vi "shag_start — 11.vi"() -> ()   [LabVIEW 2016]
uses:
  <vilib>/Instr/_visa.llb/VISA Configure Serial Port (Instr).vi
panel:
  out "положение в мин 4":i32
  out "text4":string
  out "4":i32
  out "3":i32
  out "положение в мин 3":i32
  out "text3":string
  out "text":string
  out "2":i32
  out "1":i32
  out "text2":string
  out "положение в мин 2":i32
  out "положение в мин 1":i32
  in  "all":T1(tab)
  out "положение шд 2":i32(knob) scale=-10.0..190.0
  out "текущее положение 2":string
  out "положение в минутах 2":string
  in  "Минуты 2":i32 min=-600 max=11400
  in  "Stop двигатель 2":bool
  in  "Вращение по градусам +  2":bool
  in  "Вращение по градусам -  2":bool
  in  "Вернуться в нулевое положение 2":bool
  in  "Задать текущее положение нулевым 2":bool
  in  "Установка минут 2":bool
  in  "Блокировать трубку №2":bool
  out "положение шд":i32(knob) scale=-10.0..190.0
  out "градусы минуты":string
  out "минуты":string
  in  "Минуты":i32 min=-600 max=11400
  in  "Stop двигатель":bool
  in  "Вращение по градусам +":bool
  in  "Вращение по градусам -":bool
  in  "Вернуться в нулевое положение":bool
  in  "Задать текущее положение нулевым":bool
  in  "Установка минут":bool
  in  "Блокировать зеркало №1":bool
  in  "stop":bool
  out "положение шд 3":i32(knob) scale=-10.0..190.0
  out "текущее положение 3":string
  out "положение в минутах 3":string
  in  "Минуты 3":i32 min=-600 max=11400
  in  "Stop двигатель 3":bool
  in  "Вращение по градусам +  3":bool
  in  "Вращение по градусам -  3":bool
  in  "Вернуться в нулевое положение 3":bool
  in  "Задать текущее положение нулевым 3":bool
  in  "Установка минут 3":bool
  in  "Блокировать стол №3":bool caption="Блокировать трубку №2"
  out "положение шд 4":i32(knob) scale=-10.0..190.0
  out "текущее положение 4":string
  out "положение в минутах 4":string
  in  "Минуты 4":i32 min=-600 max=11400
  in  "Stop двигатель 4":bool
  in  "Вращение по градусам +  4":bool
  in  "Вращение по градусам -  4":bool
  in  "Вернуться в нулевое положение 4":bool
  in  "Задать текущее положение нулевым 4":bool
  in  "Установка минут 4":bool
  in  "Блокировать стол №3 2":bool caption="Блокировать трубку №2"
  in  "Выберете COM порт":refnum<visa-resource-name>="COM1"
  in  "Скорость обмена данными":u32(ring)=19200 items=["9600"=9600, "19200"=19200, "38400"=38400, "57600"=57600]
  in  "Число бит на символ":u16=8 min=5 max=8 step=1
  in  "Контроль чётности":enum16{"None", "Odd", "Even", "Mark", "Space"}(ring)
  in  "Стоповый бит":u16(ring)=10 items=["1.0"=10, "1.5"=15, "2.0"=20]
  in  "Контроль переполнения":u16(ring) items=["None"=0, "XON/XOFF"=1, "RTS/CTS"=2, "DTR/DSR"=4]
  # "1 - адресс 1 двигателя\n2 - адресс 2 двигателя\n$0MV\\01+   - запуск всех двигателей в положительном направлении \n$0MS\\00   - остановка всех двигателей\n$0MJ\\04+\\00\\00\\01   - 1 шаг всех двигателей\n$0SS\\01\\10   - скорость 10 для всех двигателей"
  # "Зеркало №1"
  # "Текущее положение:"
  # "Ренгеновская трубка №2"
  # "Положение:"
  # "Поворотный стол №3"
  # "Положение:"
  # "Счётчик №4"
  # "Положение:"
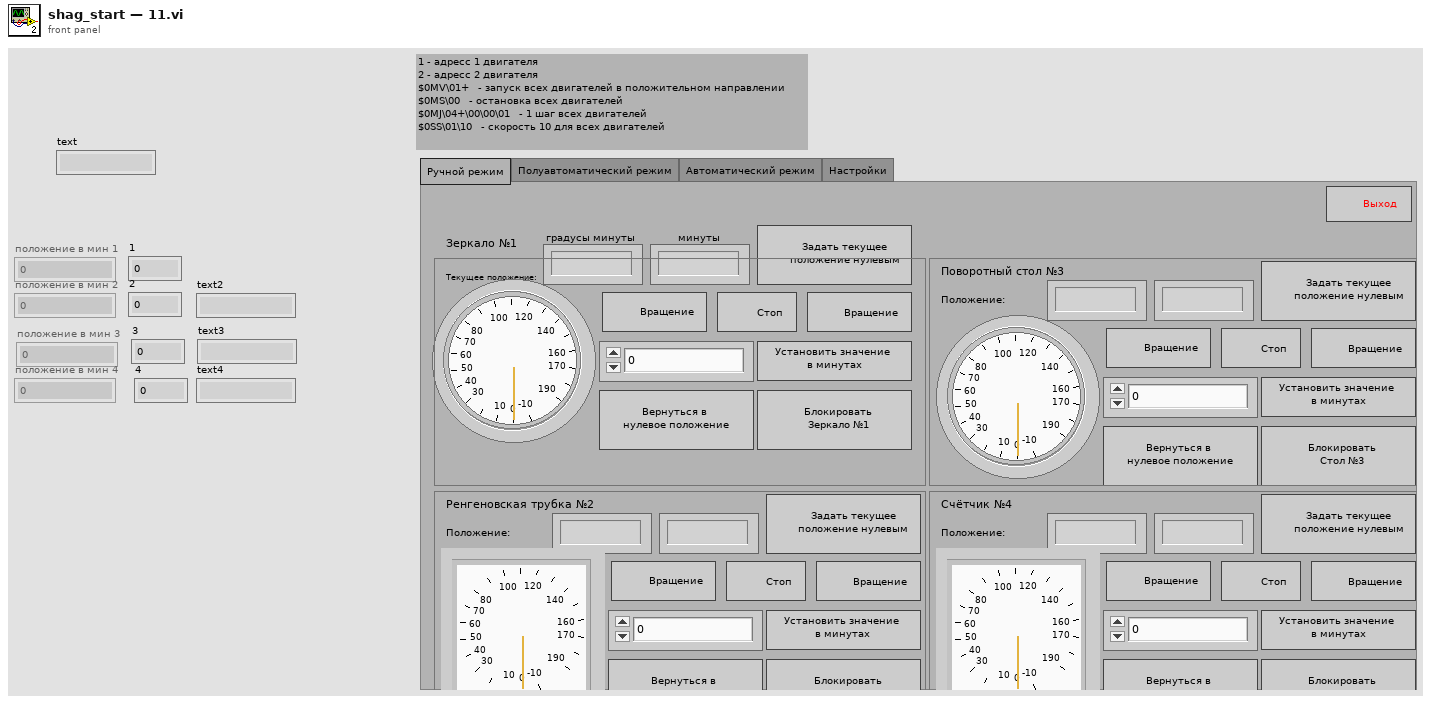
[diagram p1: front panel]
types:
  T1 = enum32{"Ручной режим", "Полуавтоматический режим", "Автоматический режим", "Настройки"}
  T2 = enum16{"open", "replace", "create", "open or create", "replace or create", "replace or create with confirmation"}
  T3 = enum8{"Enabled", "Disabled", "Disabled and Grayed Out"}
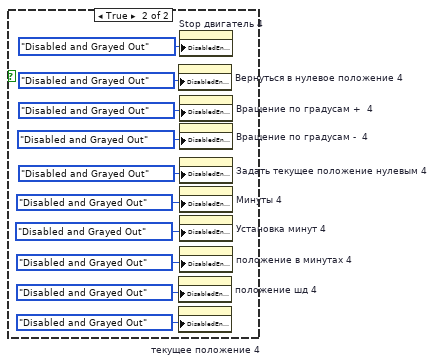
[diagram p2: hidden frame]
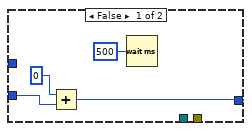
[diagram p4: hidden frame]
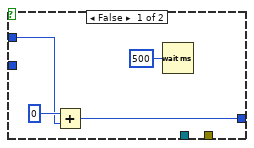
[diagram p5: hidden frame]
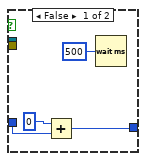
[diagram p6: hidden frame]
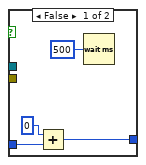
[diagram p7: hidden frame]
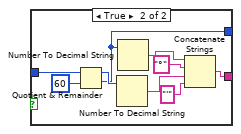
[diagram p8: hidden frame]
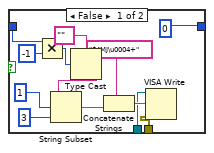
[diagram p10: hidden frame]
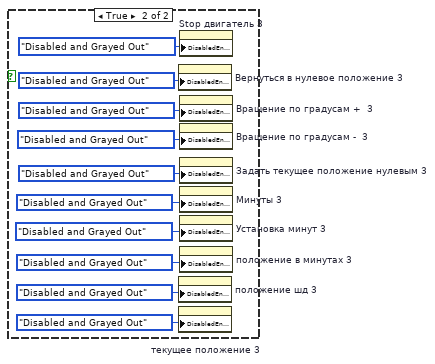
[diagram p13: hidden frame]
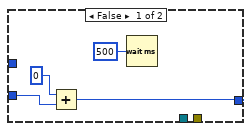
[diagram p16: hidden frame]
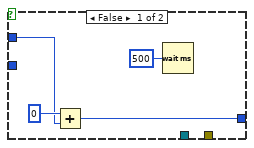
[diagram p17: hidden frame]
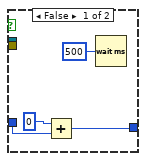
[diagram p18: hidden frame]
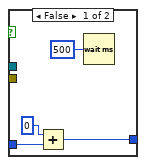
[diagram p19: hidden frame]
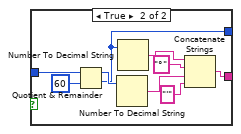
[diagram p20: hidden frame]
diagram:
  n1 = call-poly "VISA Configure Serial Port"("VISA resource name"="Выберете COM порт", "baud rate (9600)"="Скорость обмена данными", "data bits (8)"="Число бит на символ", "parity (0:none)"="Контроль чётности", "stop bits (10: 1 bit)"="Стоповый бит", "flow control (0:none)"="Контроль переполнения") -> ("VISA resource name out"=w32:refnum<visa-resource-name>, "error out"=w31:errorcluster)  [unwired: 8 in]
  n2 = Boolean To (0,1)(Boolean=FALSE ("DTR Write")) -> (0, 1=w33:i16)
  n3 = Boolean To (0,1)(Boolean=FALSE ("DTR Write")) -> (0, 1=w34:i16)
  n4 = property class="Instr"(reference=w32, error in=w31, "Serial Settings:Modem Line Settings:Line DTR State"=w33, "Serial Settings:Modem Line Settings:Line RTS State"=w34) -> (reference out=w30:refnum<visa-resource-name>, error out=w29:errorcluster)
  n5 = flat-sequence {
    tunnel: w30 -> [w63]
    tunnel: w29 -> [w62]
    tunnel: [w63] -> w28
    tunnel: [w62] -> w27
    tunnel: [w58] -> w18
    tunnel: [w66] -> w17
    tunnel: w28 -> [w66]
    tunnel: w27 -> [w65]
    tunnel: [w65] -> w15
    tunnel: [w66] -> w13
    tunnel: [w65] -> w11
    tunnel: w18 -> [w67]
    tunnel: [w65] -> w6
    tunnel: [w66] -> w5
    tunnel: [w66] -> w3
    tunnel: [w65] -> w1
    tunnel: w17 -> [w80]
    tunnel: [w80] -> w16
    tunnel: w15 -> [w79]
    tunnel: [w79] -> w14
    tunnel: w13 -> [w72]
    tunnel: [w72] -> w12
    tunnel: w11 -> [w74]
    tunnel: [w74] -> w10
    tunnel: [w75] -> w9
    tunnel: [w73] -> w8
    tunnel: [w71] -> w7
    tunnel: w6 -> [w73]
    tunnel: w5 -> [w71]
    tunnel: [w70] -> w4
    tunnel: w3 -> [w70]
    tunnel: [w69] -> w2
    tunnel: w1 -> [w69]
    tunnel: w16 -> [w90]
    tunnel: w14 -> [w89]
    tunnel: w12 -> [w85]
    tunnel: w10 -> [w88]
    tunnel: w9 -> [w87]
    tunnel: w8 -> [w84]
    tunnel: w7 -> [w83]
    tunnel: w4 -> [w82]
    tunnel: w2 -> [w81]
    frame #0 {
      n6 = VISA Write(VISA resource name=w63, write buffer="$0SS\u0001\u0010", error in (no error)=w62) -> ()  [unwired: 3 out]
      n7 = Open/Create/Replace File(file path (use dialog)=path "C:/Users/User/Desktop/shagovi_dvigatel/test_text_file", operation (0:open)=T2."open", access (0:read/write)=enum16{"read/write", "read-only", "write-only"}."read-only") -> (refnum out=w57:refnum<file>)  [unwired: 3 in, 2 out]
      n8 = Read from Text File(file (use dialog)=w57) -> (refnum out=w58:refnum<file>, text=w44:string)  [unwired: 3 in, 2 out]
      "text" <- w44
      n9 = Spreadsheet String To Array(delimiter (Tab)=" ", format string="%5f", spreadsheet string=w44) -> (array=w54:dbl[][])  [unwired: 1 in]
      n10 = Index Array(array=w54, index (row)=0 ("index")) -> (element=w52:dbl[])  [unwired: 1 in]
      n11 = Decimate 1D Array(w52) -> (w49:dbl[], w40:dbl[], w39:dbl[], w35:dbl[])
      n12 = Index Array(array=w35, index=0) -> (element=w37:dbl)
      n13 = Index Array(array=w39, index=0) -> (element=w42:dbl)
      n14 = Index Array(array=w40, index=0) -> (element=w48:dbl)
      n15 = To Long Integer(number=w37) -> (32bit integer=→"4":i32)
      n16 = To Long Integer(number=w42) -> (32bit integer=→"3":i32)
      n17 = Index Array(array=w49, index=0) -> (element=w47:dbl)
      n18 = To Long Integer(number=w48) -> (32bit integer=→"2":i32)
      n19 = To Long Integer(number=w47) -> (32bit integer=→"1":i32)
    }
    frame #1 {
      n20 = Close File(refnum=w67) -> ()  [unwired: 1 in, 2 out]
      n21 = Wait (ms)(milliseconds to wait=u32 500) -> ()  [unwired: 1 out]
    }
    frame #2 {
      n22 = Open/Create/Replace File(file path (use dialog)=path "C:/Users/User/Desktop/shagovi_dvigatel/test_text_file", operation (0:open)=T2."replace or create", access (0:read/write)=enum16{"read/write", "read-only", "write-only"}."write-only") -> (refnum out=w75:refnum<file>)  [unwired: 3 in, 2 out]
    }
    frame #3 {
      n23 = while {
        tunnel: w90 -> [w221]
        tunnel: w89 -> [w220]
        shift-right: [w216] -> _
        shift-left: _ -> [w225]
        shift-right: [w217] -> _
        shift-left: _ -> [w224]
        shift-right: [w218] -> _
        shift-left: _ -> [w223]
        shift-right: [w219] -> _
        shift-left: _ -> [w222]
        tunnel: w88 -> [w190]
        shift-right: [w212] -> w86
        shift-left: w87 -> [w213]
        tunnel: w85 -> [w189]
        shift-right: [w185] -> _
        shift-left: _ -> [w186]
        shift-right: [w183] -> _
        shift-left: _ -> [w184]
        shift-right: [w181] -> _
        shift-left: _ -> [w182]
        shift-right: [w179] -> _
        shift-left: _ -> [w180]
        tunnel: w84 -> [w157]
        tunnel: w83 -> [w156]
        shift-right: [w153] -> _
        shift-left: _ -> [w154]
        shift-right: [w151] -> _
        shift-left: _ -> [w152]
        shift-right: [w149] -> _
        shift-left: _ -> [w150]
        shift-right: [w147] -> _
        shift-left: _ -> [w148]
        tunnel: w82 -> [w125]
        tunnel: w81 -> [w124]
        shift-right: [w121] -> _
        shift-left: _ -> [w122]
        shift-right: [w119] -> _
        shift-left: _ -> [w120]
        shift-right: [w117] -> _
        shift-left: _ -> [w118]
        shift-right: [w115] -> _
        shift-left: _ -> [w116]
        stop <- "stop" stop-if-true
        # "Остановка двигателя"
        # "Управление вращением"
        # "Управление вращением"
        n24 = flat-sequence {
          tunnel: w157 -> [w549]
          tunnel: w156 -> [w548]
          tunnel: [w548] -> w178
          tunnel: [w549] -> w177
          tunnel: ["Вращение по градусам +  3"] -> w176
          tunnel: ["Вращение по градусам -  3"] -> w175
          tunnel: ["Вернуться в нулевое положение 3"] -> w174
          tunnel: ["Задать текущее положение нулевым 3"] -> w173
          tunnel: ["Установка минут 3"] -> w172
          tunnel: ["Stop двигатель 3"] -> w98
          tunnel: [w549] -> _
          tunnel: [w548] -> _
          tunnel: w178 -> [w559]
          tunnel: w177 -> [w558]
          tunnel: [w603] -> w171
          tunnel: w154 -> [w600]
          tunnel: w152 -> [w602]
          tunnel: [w601] -> w170
          tunnel: w150 -> [w599]
          tunnel: w148 -> [w598]
          tunnel: w176 -> [w584]
          tunnel: w175 -> [w583]
          tunnel: [w597] -> w169
          tunnel: [w596] -> w168
          tunnel: [w581] -> w167
          tunnel: w174 -> [w581]
          tunnel: [w558] -> w166
          tunnel: [w559] -> w165
          tunnel: [w580] -> w164
          tunnel: w173 -> [w580]
          tunnel: w172 -> [w574]
          tunnel: [w564] -> w163
          tunnel: [w557] -> w99
          tunnel: w98 -> [w557]
          tunnel: w171 -> [w689]
          tunnel: w170 -> [w690]
          tunnel: [w705] -> w162
          tunnel: [w703] -> w161
          tunnel: w169 -> [w691]
          tunnel: w168 -> [w692]
          tunnel: [w696] -> w160
          tunnel: [w701] -> w159
          tunnel: w167 -> [w699]
          tunnel: w166 -> [w695]
          tunnel: w165 -> [w694]
          tunnel: w164 -> [w693]
          tunnel: [w693] -> w158
          tunnel: w163 -> [w680]
          tunnel: [w673] -> w100
          tunnel: w99 -> [w673]
          tunnel: [w787] -> w153
          tunnel: [w784] -> w151
          tunnel: w162 -> [w786]
          tunnel: w161 -> [w785]
          tunnel: [w783] -> w149
          tunnel: [w782] -> w147
          tunnel: w160 -> [w781]
          tunnel: w159 -> [w780]
          tunnel: w158 -> [w778]
          tunnel: w100 -> [w777]
          frame #0 {
            n25 = Wait Until Next ms Multiple(millisecond multiple=u32 500) -> ()  [unwired: 1 out]
          }
          frame #1 {
            n26 = Greater?(x="Минуты 3", y=0) -> (0:w572:bool)
            n27 = Not Equal?(x="Минуты 3", y=0) -> (x != y?=w571:bool)
            n28 = local read "положение в мин 3"() -> (w565:i32)
            n29 = Add(x="Минуты 3", y=w565) -> (x+y=w594:i32)
            n30 = Add(x="Минуты 3", y=w565) -> (x+y=w567:i32)
            n31 = Not Equal?(x="Минуты 3", y=0) -> (x != y?=w569:bool)
            n32 = Add(x=w565, y=60) -> (x+y=w589:i32)
            n33 = Subtract(x=w565, y=60) -> (x-y=w577:i32)
            n34 = Not(x=w572) -> (.not. x?=w573:bool)
            n35 = Greater Or Equal?(x=w567, y=-600) -> (x >= y?=w568:bool)
            n36 = Less Or Equal?(x=w594, y=11400) -> (x <= y?=w570:bool)
            n37 = Less Or Equal?(x=w589, y=11390) -> (x <= y?=w586:bool)
            n38 = Greater Or Equal?(x=w577, y=-590) -> (x >= y?=w578:bool)
            n39 = Compound Arithmetic op=AND(w573, w569, w568) -> (w590:bool)
            n40 = And(x=w584, y=w586) -> (x .and. y?=w585:bool)
            n41 = And(x=w583, y=w578) -> (x .and. y?=w582:bool)
            n42 = Compound Arithmetic op=AND(w572, w571, w570) -> (w592:bool)
            n43 = case shown="True" w574 {
              tunnel: [w609 w618] -> w603
              tunnel: w602 -> [w608 w617]
              tunnel: [w608 w616] -> w601
              tunnel: w600 -> [w609 w615]
              tunnel: w592 -> [_ w614]
              tunnel: w590 -> [_ w613]
              tunnel: w558 -> [_ w612]
              tunnel: w559 -> [_ w611]
              tunnel: "Минуты 3" -> [_ w610]
              frame False {
              }
              frame True {
                n44 = case shown="True" w614 {
                  tunnel: [w639 w645] -> w618
                  tunnel: w615 -> [w638 w644]
                  tunnel: w612 -> [_ w643]
                  tunnel: w611 -> [_ w642]
                  tunnel: w610 -> [_ w641]
                  frame False {
                    n45 = Add(x=0, y=w638) -> (x+y=w639:i32)
                    n46 = Wait (ms)(milliseconds to wait=u32 500) -> ()  [unwired: 1 out]
                  }
                  frame True {
                    n47 = Type Cast(type="", x=w641) -> (*(type *) &x=w648:string)
                    n48 = Add(x=w641, y=w644) -> (x+y=w645:i32)
                    n49 = String Subset(string=w648, offset (0)=1, length (rest)=3 ("length (rest)")) -> (substring=w647:string)
                    n50 = Concatenate Strings("$3MJ\u0004+" ("write buffer"), w647) -> (w651:string)
                    n51 = VISA Write(VISA resource name=w642, write buffer=w651, error in (no error)=w643) -> ()  [unwired: 3 out]
                  }
                }
                n52 = case shown="True" w613 {
                  tunnel: [w621 w627] -> w616
                  tunnel: w617 -> [w620 w626]
                  tunnel: w611 -> [_ w629]
                  tunnel: w612 -> [_ w628]
                  tunnel: w610 -> [_ w623]
                  frame False {
                    n53 = Add(x=0, y=w620) -> (x+y=w621:i32)
                    n54 = Wait (ms)(milliseconds to wait=u32 500) -> ()  [unwired: 1 out]
                  }
                  frame True {
                    n55 = Multiply(x=w623, y=-1) -> (x*y=w625:i32)
                    n56 = Type Cast(type="", x=w625) -> (*(type *) &x=w632:string)
                    n57 = Add(x=w626, y=w623) -> (x+y=w627:i32)
                    n58 = String Subset(string=w632, offset (0)=1, length (rest)=3 ("length (rest)")) -> (substring=w631:string)
                    n59 = Concatenate Strings("$3MJ\u0004-" ("write buffer"), w631) -> (w635:string)
                    n60 = VISA Write(VISA resource name=w629, write buffer=w635, error in (no error)=w628) -> ()  [unwired: 3 out]
                  }
                }
              }
            }
            n61 = case shown="True" w585 {
              tunnel: [w665 w672] -> w597
              tunnel: w599 -> [w664 w667]
              tunnel: w559 -> [_ w668]
              tunnel: w558 -> [_ w669]
              frame False {
                n62 = Add(x=0, y=w664) -> (x+y=w665:i32)
                n63 = Wait (ms)(milliseconds to wait=u32 500) -> ()  [unwired: 1 out]
              }
              frame True {
                n64 = VISA Write(VISA resource name=w668, write buffer="$3MJ\u0004+\u0000\u0000<", error in (no error)=w669) -> ()  [unwired: 3 out]
                n65 = Add(x=60, y=w667) -> (x+y=w672:i32)
              }
            }
            n66 = case shown="True" w582 {
              tunnel: [w655 w658] -> w596
              tunnel: w598 -> [w654 w657]
              tunnel: w559 -> [_ w661]
              tunnel: w558 -> [_ w660]
              frame False {
                n67 = Add(x=0, y=w654) -> (x+y=w655:i32)
                n68 = Wait (ms)(milliseconds to wait=u32 500) -> ()  [unwired: 1 out]
              }
              frame True {
                n69 = Subtract(x=w657, y=60 ("x")) -> (x-y=w658:i32)
                n70 = VISA Write(VISA resource name=w661, write buffer="$3MJ\u0004-\u0000\u0000<", error in (no error)=w660) -> ()  [unwired: 3 out]
              }
            }
            n71 = for {
              N: 1 -> [_]
              tunnel: [w607] -> w562 mode=indexing
              n72 = local read "3"() -> (w607:i32)
            }
            n73 = case shown="True" w557 {
              tunnel: w559 -> [_ w605]
              tunnel: w558 -> [_ w604]
              frame False {
              }
              frame True {
                n74 = VISA Write(VISA resource name=w605, write buffer="$3MS\u0001", error in (no error)=w604) -> ()  [unwired: 3 out]
              }
            }
            n75 = Index Array(array=w562, index=0) -> (element=w564:i32)
          }
          frame #2 {
            # "Нулевое положение"
            n76 = Add(x=w691, y=w692) -> (x+y=w700:i32)
            n77 = Add(x=w689, y=w690) -> (x+y=w702:i32)
            n78 = Add(x=w702, y=w700) -> (x+y=w685:i32)
            n79 = Add(x=w685, y=w680) -> (x+y=w684:i32)
            n80 = Not Equal?(x=w684, y=0 ("x")) -> (x != y?=w697:bool)
            n81 = And(x=w697, y=w699) -> (x .and. y?=w704:bool)
            n82 = case shown="True" w704 {
              tunnel: [w729 w752] -> w676
              tunnel: w689 -> [w733 w749]
              tunnel: [w733 w748] -> w705
              tunnel: [w732 w747] -> w703
              tunnel: w684 -> [w729 w741]
              tunnel: [w730 w743] -> w701
              tunnel: [w731 w740] -> w696
              tunnel: w690 -> [w732 w739]
              tunnel: w695 -> [_ w738]
              tunnel: w694 -> [_ w737]
              tunnel: w691 -> [w731 w736]
              tunnel: w692 -> [w730 w735]
              frame False {
              }
              frame True {
                n83 = Greater?(x=w741, y=0) -> (0:w742:bool)
                n84 = Multiply(x=w735, y=0) -> (x*y=w743:i32)
                n85 = Multiply(x=w739, y=0) -> (x*y=w747:i32)
                n86 = case shown="False" w742 {
                  tunnel: w741 -> [w757 w770]
                  tunnel: [0 0] -> w752
                  tunnel: w737 -> [w754 w767]
                  tunnel: w738 -> [w753 w766]
                  frame False {
                    n87 = Multiply(x=w757, y=-1) -> (x*y=w755:i32)
                    n88 = Type Cast(type="", x=w755) -> (*(type *) &x=w761:string)
                    n89 = String Subset(string=w761, offset (0)=1, length (rest)=3 ("length (rest)")) -> (substring=w760:string)
                    n90 = Concatenate Strings("$3MJ\u0004+" ("write buffer"), w760) -> (w764:string)
                    n91 = VISA Write(VISA resource name=w754, write buffer=w764, error in (no error)=w753) -> ()  [unwired: 3 out]
                  }
                  frame True {
                    n92 = Type Cast(type="", x=w770) -> (*(type *) &x=w773:string)
                    n93 = String Subset(string=w773, offset (0)=1, length (rest)=3 ("length (rest)")) -> (substring=w772:string)
                    n94 = Concatenate Strings("$3MJ\u0004-" ("write buffer"), w772) -> (w768:string)
                    n95 = VISA Write(VISA resource name=w767, write buffer=w768, error in (no error)=w766) -> ()  [unwired: 3 out]
                  }
                }
                n96 = local write "3"(0 ("3")) -> ()
                n97 = Multiply(x=w736, y=0) -> (x*y=w740:i32)
                n98 = Multiply(x=w749, y=0) -> (x*y=w748:i32)
              }
            }
            "положение в мин 3" <- w676
            n99 = Greater Or Equal?(x=w676, y=0) -> (x >= y?=w674:bool)
            n100 = Number To Decimal String(number=w676, width (-)=i16 1) -> (decimal integer string=w687:string)
            n101 = case shown="False" w674 {
              tunnel: w676 -> [w712 w728]
              tunnel: [w716 w722] -> w679
              tunnel: [w706 w720] -> w677
              frame False {
                n102 = Multiply(x=-1, y=w712) -> (x*y=w711:i32)
                n103 = Quotient & Remainder(x=w711, y=60) -> (x-y*floor(x/y)=w715:i32, floor(x/y)=w707:i32)
                n104 = Multiply(x=-1, y=w707) -> (x*y=w706:i32)
                n105 = Number To Decimal String(number=w707) -> (decimal integer string=w713:string)  [unwired: 1 in]
                n106 = Number To Decimal String(number=w715) -> (decimal integer string=w714:string)  [unwired: 1 in]
                n107 = Concatenate Strings("-" ("string"), w713, "°" ("string"), w714, "'" ("string")) -> (w716:string)
              }
              frame True {
                n108 = Quotient & Remainder(x=w728, y=60) -> (x-y*floor(x/y)=w721:i32, floor(x/y)=w720:i32)
                n109 = Number To Decimal String(number=w721) -> (decimal integer string=w723:string)  [unwired: 1 in]
                n110 = Number To Decimal String(number=w720) -> (decimal integer string=w724:string)  [unwired: 1 in]
                n111 = Concatenate Strings(w724, "°" ("string"), w723, "'" ("string")) -> (w722:string)
              }
            }
            "текущее положение 3" <- w679
            "положение шд 3" <- w677
            n112 = Concatenate Strings(w687, "'" ("string")) -> (→"положение в минутах 3":string)
            n113 = Format Into String(w676) -> (resulting string=w682:string)  [unwired: 3 in, 1 out]
            n114 = call <vilib>:"Space Constant.vi"() -> ("String"=w681:string)
            n115 = Concatenate Strings(w681, w682) -> (→"text3":string)
          }
          frame #3 {
            # "Задача нуля"
            n116 = Or(x=w777, y=w778) -> (x .or. y?=w779:bool)
            n117 = case shown="True" w779 {
              tunnel: [w791 w803] -> w787
              tunnel: w786 -> [w791 w804]
              tunnel: w785 -> [w790 w800]
              tunnel: [w790 w799] -> w784
              tunnel: [w789 w796] -> w783
              tunnel: [w788 w795] -> w782
              tunnel: w781 -> [w789 w794]
              tunnel: w780 -> [w788 w793]
              frame False {
              }
              frame True {
                n118 = Multiply(x=w800, y=0) -> (x*y=w799:i32)
                n119 = Multiply(x=w804, y=0) -> (x*y=w803:i32)
                n120 = Multiply(x=w793, y=0) -> (x*y=w795:i32)
                n121 = Multiply(x=w794, y=0) -> (x*y=w796:i32)
                n122 = local write "3"(0 ("3")) -> ()
              }
            }
          }
        }
        n123 = flat-sequence {
          tunnel: w190 -> [w832]
          tunnel: w189 -> [w833]
          tunnel: [w833] -> w211
          tunnel: [w832] -> w210
          tunnel: ["Вращение по градусам +  2"] -> w209
          tunnel: ["Вращение по градусам -  2"] -> w208
          tunnel: ["Вернуться в нулевое положение 2"] -> w207
          tunnel: ["Задать текущее положение нулевым 2"] -> w206
          tunnel: ["Установка минут 2"] -> w205
          tunnel: ["Stop двигатель 2"] -> w105
          tunnel: w211 -> [w834]
          tunnel: w210 -> [w835]
          tunnel: [w880] -> w204
          tunnel: w186 -> [w877]
          tunnel: w184 -> [w879]
          tunnel: [w878] -> w203
          tunnel: w182 -> [w876]
          tunnel: w180 -> [w875]
          tunnel: w209 -> [w861]
          tunnel: w208 -> [w860]
          tunnel: [w874] -> w202
          tunnel: [w873] -> w201
          tunnel: [w858] -> w200
          tunnel: w207 -> [w858]
          tunnel: [w835] -> w199
          tunnel: [w834] -> w198
          tunnel: [w857] -> w197
          tunnel: w206 -> [w857]
          tunnel: w205 -> [w851]
          tunnel: [w841] -> w196
          tunnel: [w836] -> w106
          tunnel: w105 -> [w836]
          tunnel: [w835] -> w103
          tunnel: [w834] -> w102
          tunnel: w204 -> [w965]
          tunnel: w203 -> [w966]
          tunnel: [w981] -> w195
          tunnel: [w979] -> w194
          tunnel: w202 -> [w967]
          tunnel: w201 -> [w968]
          tunnel: [w972] -> w193
          tunnel: [w977] -> w192
          tunnel: w200 -> [w975]
          tunnel: w199 -> [w971]
          tunnel: w198 -> [w970]
          tunnel: w197 -> [w969]
          tunnel: [w969] -> w191
          tunnel: w196 -> [w953]
          tunnel: [w949] -> w107
          tunnel: w106 -> [w949]
          tunnel: [w948] -> w104
          tunnel: w103 -> [w948]
          tunnel: w102 -> [w947]
          tunnel: [w947] -> w101
          tunnel: [w1065] -> w185
          tunnel: [w1062] -> w183
          tunnel: w195 -> [w1064]
          tunnel: w194 -> [w1063]
          tunnel: [w1061] -> w181
          tunnel: [w1060] -> w179
          tunnel: w193 -> [w1059]
          tunnel: w192 -> [w1058]
          tunnel: w191 -> [w1057]
          tunnel: w107 -> [w1055]
          tunnel: w104 -> [w1054]
          tunnel: w101 -> [w1053]
          frame #0 {
            n124 = Wait Until Next ms Multiple(millisecond multiple=u32 300) -> ()  [unwired: 1 out]
          }
          frame #1 {
            n125 = Greater?(x="Минуты 2", y=0) -> (0:w849:bool)
            n126 = Not Equal?(x="Минуты 2", y=0) -> (x != y?=w848:bool)
            n127 = local read "положение в мин 2"() -> (w842:i32)
            n128 = Add(x="Минуты 2", y=w842) -> (x+y=w871:i32)
            n129 = Add(x="Минуты 2", y=w842) -> (x+y=w844:i32)
            n130 = Not Equal?(x="Минуты 2", y=0) -> (x != y?=w846:bool)
            n131 = Add(x=w842, y=60) -> (x+y=w866:i32)
            n132 = Subtract(x=w842, y=60) -> (x-y=w854:i32)
            n133 = Not(x=w849) -> (.not. x?=w850:bool)
            n134 = Greater Or Equal?(x=w844, y=-600) -> (x >= y?=w845:bool)
            n135 = Less Or Equal?(x=w871, y=11400) -> (x <= y?=w847:bool)
            n136 = Less Or Equal?(x=w866, y=11390) -> (x <= y?=w863:bool)
            n137 = Greater Or Equal?(x=w854, y=-590) -> (x >= y?=w855:bool)
            n138 = Compound Arithmetic op=AND(w850, w846, w845) -> (w867:bool)
            n139 = And(x=w861, y=w863) -> (x .and. y?=w862:bool)
            n140 = And(x=w860, y=w855) -> (x .and. y?=w859:bool)
            n141 = Compound Arithmetic op=AND(w849, w848, w847) -> (w869:bool)
            n142 = case shown="True" w851 {
              tunnel: [w883 w892] -> w880
              tunnel: w879 -> [w882 w891]
              tunnel: [w882 w890] -> w878
              tunnel: w877 -> [w883 w889]
              tunnel: w869 -> [_ w888]
              tunnel: w867 -> [_ w887]
              tunnel: w835 -> [_ w886]
              tunnel: w834 -> [_ w885]
              tunnel: "Минуты 2" -> [_ w884]
              frame False {
              }
              frame True {
                n143 = case shown="True" w888 {
                  tunnel: [w913 w919] -> w892
                  tunnel: w889 -> [w912 w918]
                  tunnel: w886 -> [_ w917]
                  tunnel: w885 -> [_ w916]
                  tunnel: w884 -> [_ w915]
                  frame False {
                    n144 = Add(x=0, y=w912) -> (x+y=w913:i32)
                    n145 = Wait (ms)(milliseconds to wait=u32 500) -> ()  [unwired: 1 out]
                  }
                  frame True {
                    n146 = Type Cast(type="", x=w915) -> (*(type *) &x=w922:string)
                    n147 = Add(x=w915, y=w918) -> (x+y=w919:i32)
                    n148 = String Subset(string=w922, offset (0)=1, length (rest)=3 ("length (rest)")) -> (substring=w921:string)
                    n149 = Concatenate Strings("$2MJ\u0004+" ("write buffer"), w921) -> (w925:string)
                    n150 = VISA Write(VISA resource name=w916, write buffer=w925, error in (no error)=w917) -> ()  [unwired: 3 out]
                  }
                }
                n151 = case shown="True" w887 {
                  tunnel: [w895 w901] -> w890
                  tunnel: w891 -> [w894 w900]
                  tunnel: w885 -> [_ w903]
                  tunnel: w886 -> [_ w902]
                  tunnel: w884 -> [_ w897]
                  frame False {
                    n152 = Add(x=0, y=w894) -> (x+y=w895:i32)
                    n153 = Wait (ms)(milliseconds to wait=u32 500) -> ()  [unwired: 1 out]
                  }
                  frame True {
                    n154 = Multiply(x=w897, y=-1) -> (x*y=w899:i32)
                    n155 = Type Cast(type="", x=w899) -> (*(type *) &x=w906:string)
                    n156 = Add(x=w900, y=w897) -> (x+y=w901:i32)
                    n157 = String Subset(string=w906, offset (0)=1, length (rest)=3 ("length (rest)")) -> (substring=w905:string)
                    n158 = Concatenate Strings("$2MJ\u0004-" ("write buffer"), w905) -> (w909:string)
                    n159 = VISA Write(VISA resource name=w903, write buffer=w909, error in (no error)=w902) -> ()  [unwired: 3 out]
                  }
                }
              }
            }
            n160 = case shown="True" w862 {
              tunnel: [w939 w946] -> w874
              tunnel: w876 -> [w938 w941]
              tunnel: w834 -> [_ w942]
              tunnel: w835 -> [_ w943]
              frame False {
                n161 = Add(x=0, y=w938) -> (x+y=w939:i32)
                n162 = Wait (ms)(milliseconds to wait=u32 500) -> ()  [unwired: 1 out]
              }
              frame True {
                n163 = VISA Write(VISA resource name=w942, write buffer="$2MJ\u0004+\u0000\u0000<", error in (no error)=w943) -> ()  [unwired: 3 out]
                n164 = Add(x=60, y=w941) -> (x+y=w946:i32)
              }
            }
            n165 = case shown="True" w859 {
              tunnel: [w929 w932] -> w873
              tunnel: w875 -> [w928 w931]
              tunnel: w834 -> [_ w935]
              tunnel: w835 -> [_ w934]
              frame False {
                n166 = Add(x=0, y=w928) -> (x+y=w929:i32)
                n167 = Wait (ms)(milliseconds to wait=u32 500) -> ()  [unwired: 1 out]
              }
              frame True {
                n168 = Subtract(x=w931, y=60 ("x")) -> (x-y=w932:i32)
                n169 = VISA Write(VISA resource name=w935, write buffer="$2MJ\u0004-\u0000\u0000<", error in (no error)=w934) -> ()  [unwired: 3 out]
              }
            }
            n170 = for {
              N: 1 -> [_]
              tunnel: [w881] -> w839 mode=indexing
              n171 = local read "2"() -> (w881:i32)
            }
            n172 = Index Array(array=w839, index=0) -> (element=w841:i32)
          }
          frame #2 {
            # "Нулевое положение"
            n173 = Add(x=w967, y=w968) -> (x+y=w976:i32)
            n174 = Add(x=w965, y=w966) -> (x+y=w978:i32)
            n175 = Add(x=w978, y=w976) -> (x+y=w961:i32)
            n176 = Add(x=w961, y=w953) -> (x+y=w960:i32)
            n177 = Not Equal?(x=w960, y=0 ("x")) -> (x != y?=w973:bool)
            n178 = And(x=w973, y=w975) -> (x .and. y?=w980:bool)
            n179 = case shown="True" w980 {
              tunnel: [w1005 w1028] -> w952
              tunnel: w965 -> [w1009 w1025]
              tunnel: [w1009 w1024] -> w981
              tunnel: [w1008 w1023] -> w979
              tunnel: w960 -> [w1005 w1017]
              tunnel: [w1006 w1019] -> w977
              tunnel: [w1007 w1016] -> w972
              tunnel: w966 -> [w1008 w1015]
              tunnel: w971 -> [_ w1014]
              tunnel: w970 -> [_ w1013]
              tunnel: w967 -> [w1007 w1012]
              tunnel: w968 -> [w1006 w1011]
              frame False {
              }
              frame True {
                n180 = Greater?(x=w1017, y=0) -> (0:w1018:bool)
                n181 = Multiply(x=w1011, y=0) -> (x*y=w1019:i32)
                n182 = Multiply(x=w1015, y=0) -> (x*y=w1023:i32)
                n183 = case shown="True" w1018 {
                  tunnel: w1017 -> [w1033 w1046]
                  tunnel: [0 0] -> w1028
                  tunnel: w1013 -> [w1030 w1043]
                  tunnel: w1014 -> [w1029 w1042]
                  frame False {
                    n184 = Multiply(x=w1033, y=-1) -> (x*y=w1031:i32)
                    n185 = Type Cast(type="", x=w1031) -> (*(type *) &x=w1037:string)
                    n186 = String Subset(string=w1037, offset (0)=1, length (rest)=3 ("length (rest)")) -> (substring=w1036:string)
                    n187 = Concatenate Strings("$2MJ\u0004+" ("write buffer"), w1036) -> (w1040:string)
                    n188 = VISA Write(VISA resource name=w1030, write buffer=w1040, error in (no error)=w1029) -> ()  [unwired: 3 out]
                  }
                  frame True {
                    n189 = Type Cast(type="", x=w1046) -> (*(type *) &x=w1049:string)
                    n190 = String Subset(string=w1049, offset (0)=1, length (rest)=3 ("length (rest)")) -> (substring=w1048:string)
                    n191 = Concatenate Strings("$2MJ\u0004-" ("write buffer"), w1048) -> (w1044:string)
                    n192 = VISA Write(VISA resource name=w1043, write buffer=w1044, error in (no error)=w1042) -> ()  [unwired: 3 out]
                  }
                }
                n193 = Multiply(x=w1012, y=0) -> (x*y=w1016:i32)
                n194 = local write "2"(0 ("2")) -> ()
                n195 = Multiply(x=w1025, y=0) -> (x*y=w1024:i32)
              }
            }
            "положение в мин 2" <- w952
            n196 = Greater Or Equal?(x=w952, y=0) -> (x >= y?=w951:bool)
            n197 = Number To Decimal String(number=w952, width (-)=i16 1) -> (decimal integer string=w963:string)
            n198 = case shown="False" w951 {
              tunnel: w952 -> [w988 w1004]
              tunnel: [w992 w998] -> w958
              tunnel: [w982 w996] -> w957
              frame False {
                n199 = Multiply(x=-1, y=w988) -> (x*y=w987:i32)
                n200 = Quotient & Remainder(x=w987, y=60) -> (x-y*floor(x/y)=w991:i32, floor(x/y)=w983:i32)
                n201 = Multiply(x=-1, y=w983) -> (x*y=w982:i32)
                n202 = Number To Decimal String(number=w983) -> (decimal integer string=w989:string)  [unwired: 1 in]
                n203 = Number To Decimal String(number=w991) -> (decimal integer string=w990:string)  [unwired: 1 in]
                n204 = Concatenate Strings("-" ("string"), w989, "°" ("string"), w990, "'" ("string")) -> (w992:string)
              }
              frame True {
                n205 = Quotient & Remainder(x=w1004, y=60) -> (x-y*floor(x/y)=w997:i32, floor(x/y)=w996:i32)
                n206 = Number To Decimal String(number=w997) -> (decimal integer string=w999:string)  [unwired: 1 in]
                n207 = Number To Decimal String(number=w996) -> (decimal integer string=w1000:string)  [unwired: 1 in]
                n208 = Concatenate Strings(w1000, "°" ("string"), w999, "'" ("string")) -> (w998:string)
              }
            }
            "положение шд 2" <- w957
            "текущее положение 2" <- w958
            n209 = Concatenate Strings(w963, "'" ("string")) -> (→"положение в минутах 2":string)
            n210 = Format Into String(w952) -> (resulting string=w955:string)  [unwired: 3 in, 1 out]
            n211 = call <vilib>:"Space Constant.vi"() -> ("String"=w954:string)
            n212 = Concatenate Strings(w954, w955) -> (→"text2":string)
          }
          frame #3 {
            # "Остановка двигателя"
            # "Задача нуля"
            n213 = Or(x=w1055, y=w1057) -> (x .or. y?=w1056:bool)
            n214 = case shown="True" w1056 {
              tunnel: [w1073 w1085] -> w1065
              tunnel: w1064 -> [w1073 w1086]
              tunnel: w1063 -> [w1072 w1082]
              tunnel: [w1072 w1081] -> w1062
              tunnel: [w1071 w1078] -> w1061
              tunnel: [w1070 w1077] -> w1060
              tunnel: w1059 -> [w1071 w1076]
              tunnel: w1058 -> [w1070 w1075]
              frame False {
              }
              frame True {
                n215 = Multiply(x=w1082, y=0) -> (x*y=w1081:i32)
                n216 = Multiply(x=w1086, y=0) -> (x*y=w1085:i32)
                n217 = Multiply(x=w1075, y=0) -> (x*y=w1077:i32)
                n218 = Multiply(x=w1076, y=0) -> (x*y=w1078:i32)
                n219 = local write "2"(0 ("2")) -> ()
              }
            }
            n220 = case shown="True" w1055 {
              tunnel: w1053 -> [_ w1067]
              tunnel: w1054 -> [_ w1066]
              frame False {
              }
              frame True {
                n221 = Wait (ms)(milliseconds to wait=u32 500) -> ()  [unwired: 1 out]
                n222 = VISA Write(VISA resource name=w1067, write buffer="$2MS\u0001", error in (no error)=w1066) -> ()  [unwired: 3 out]
              }
            }
          }
        }
        n223 = flat-sequence {
          tunnel: w220 -> [w1114]
          tunnel: w221 -> [w1115]
          tunnel: [w1115] -> w245
          tunnel: [w1114] -> w244
          tunnel: ["Вращение по градусам +"] -> w243
          tunnel: ["Вращение по градусам -"] -> w242
          tunnel: ["Вернуться в нулевое положение"] -> w241
          tunnel: ["Задать текущее положение нулевым"] -> w240
          tunnel: ["Установка минут"] -> w239
          tunnel: ["Stop двигатель"] -> w114
          tunnel: w245 -> [w1117]
          tunnel: w244 -> [w1116]
          tunnel: [w1162] -> w238
          tunnel: w225 -> [w1159]
          tunnel: w224 -> [w1161]
          tunnel: [w1160] -> w237
          tunnel: w223 -> [w1158]
          tunnel: w222 -> [w1157]
          tunnel: w243 -> [w1143]
          tunnel: w242 -> [w1142]
          tunnel: [w1156] -> w236
          tunnel: [w1155] -> w235
          tunnel: [w1140] -> w234
          tunnel: w241 -> [w1140]
          tunnel: [w1116] -> w233
          tunnel: [w1117] -> w232
          tunnel: [w1139] -> w231
          tunnel: w240 -> [w1139]
          tunnel: w239 -> [w1133]
          tunnel: [w1122] -> w214
          tunnel: w114 -> [w1118]
          tunnel: [w1118] -> w112
          tunnel: [w1117] -> w111
          tunnel: [w1116] -> w109
          tunnel: w238 -> [w1245]
          tunnel: w237 -> [w1246]
          tunnel: [w1263] -> w230
          tunnel: [w1261] -> w229
          tunnel: w236 -> [w1247]
          tunnel: w235 -> [w1248]
          tunnel: [w1254] -> w228
          tunnel: [w1259] -> w227
          tunnel: w234 -> [w1257]
          tunnel: w233 -> [w1253]
          tunnel: w232 -> [w1252]
          tunnel: w231 -> [w1250]
          tunnel: [w1250] -> w226
          tunnel: [w1239] -> _
          tunnel: "stop" -> [w1242]
          tunnel: w213 -> [w1239]
          tunnel: w214 -> [w1235]
          tunnel: [w1236] -> w212
          tunnel: [w1231] -> w113
          tunnel: w112 -> [w1231]
          tunnel: w111 -> [w1230]
          tunnel: [w1230] -> w110
          tunnel: w109 -> [w1229]
          tunnel: [w1229] -> w108
          tunnel: [w1356] -> w216
          tunnel: [w1353] -> w217
          tunnel: w230 -> [w1355]
          tunnel: w229 -> [w1354]
          tunnel: [w1352] -> w218
          tunnel: [w1351] -> w219
          tunnel: w228 -> [w1350]
          tunnel: w227 -> [w1349]
          tunnel: w226 -> [w1346]
          tunnel: w113 -> [w1345]
          tunnel: w110 -> [w1348]
          tunnel: w108 -> [w1347]
          frame #0 {
            n224 = Wait Until Next ms Multiple(millisecond multiple=u32 300) -> ()  [unwired: 1 out]
          }
          frame #1 {
            n225 = Greater?(x="Минуты", y=0) -> (0:w1131:bool)
            n226 = Not Equal?(x="Минуты", y=0) -> (x != y?=w1130:bool)
            n227 = local read "положение в мин 1"() -> (w1123:i32)
            n228 = Add(x="Минуты", y=w1123) -> (x+y=w1153:i32)
            n229 = Add(x="Минуты", y=w1123) -> (x+y=w1125:i32)
            n230 = Not Equal?(x="Минуты", y=0) -> (x != y?=w1128:bool)
            n231 = Add(x=w1123, y=60) -> (x+y=w1148:i32)
            n232 = Subtract(x=w1123, y=60) -> (x-y=w1136:i32)
            n233 = Not(x=w1131) -> (.not. x?=w1132:bool)
            n234 = Greater Or Equal?(x=w1125, y=-600) -> (x >= y?=w1126:bool)
            n235 = Less Or Equal?(x=w1153, y=11400) -> (x <= y?=w1129:bool)
            n236 = Less Or Equal?(x=w1148, y=11390) -> (x <= y?=w1145:bool)
            n237 = Greater Or Equal?(x=w1136, y=-590) -> (x >= y?=w1137:bool)
            n238 = Compound Arithmetic op=AND(w1132, w1128, w1126) -> (w1149:bool)
            n239 = And(x=w1143, y=w1145) -> (x .and. y?=w1144:bool)
            n240 = And(x=w1142, y=w1137) -> (x .and. y?=w1141:bool)
            n241 = Compound Arithmetic op=AND(w1131, w1130, w1129) -> (w1151:bool)
            n242 = case shown="True" w1133 {
              tunnel: [w1165 w1174] -> w1162
              tunnel: w1161 -> [w1164 w1173]
              tunnel: [w1164 w1172] -> w1160
              tunnel: w1159 -> [w1165 w1171]
              tunnel: w1151 -> [_ w1170]
              tunnel: w1149 -> [_ w1169]
              tunnel: w1116 -> [_ w1168]
              tunnel: w1117 -> [_ w1167]
              tunnel: "Минуты" -> [_ w1166]
              frame False {
              }
              frame True {
                n243 = case shown="True" w1170 {
                  tunnel: [w1195 w1201] -> w1174
                  tunnel: w1171 -> [w1194 w1200]
                  tunnel: w1168 -> [_ w1199]
                  tunnel: w1167 -> [_ w1198]
                  tunnel: w1166 -> [_ w1197]
                  frame False {
                    n244 = Add(x=0, y=w1194) -> (x+y=w1195:i32)
                    n245 = Wait (ms)(milliseconds to wait=u32 500) -> ()  [unwired: 1 out]
                  }
                  frame True {
                    n246 = Type Cast(type="", x=w1197) -> (*(type *) &x=w1204:string)
                    n247 = Add(x=w1197, y=w1200) -> (x+y=w1201:i32)
                    n248 = String Subset(string=w1204, offset (0)=1, length (rest)=3 ("length (rest)")) -> (substring=w1203:string)
                    n249 = Concatenate Strings("$1MJ\u0004+" ("write buffer"), w1203) -> (w1207:string)
                    n250 = VISA Write(VISA resource name=w1198, write buffer=w1207, error in (no error)=w1199) -> ()  [unwired: 3 out]
                  }
                }
                n251 = case shown="True" w1169 {
                  tunnel: [w1177 w1183] -> w1172
                  tunnel: w1173 -> [w1176 w1182]
                  tunnel: w1167 -> [_ w1185]
                  tunnel: w1168 -> [_ w1184]
                  tunnel: w1166 -> [_ w1179]
                  frame False {
                    n252 = Add(x=0, y=w1176) -> (x+y=w1177:i32)
                    n253 = Wait (ms)(milliseconds to wait=u32 500) -> ()  [unwired: 1 out]
                  }
                  frame True {
                    n254 = Multiply(x=w1179, y=-1) -> (x*y=w1181:i32)
                    n255 = Type Cast(type="", x=w1181) -> (*(type *) &x=w1188:string)
                    n256 = Add(x=w1182, y=w1179) -> (x+y=w1183:i32)
                    n257 = String Subset(string=w1188, offset (0)=1, length (rest)=3 ("length (rest)")) -> (substring=w1187:string)
                    n258 = Concatenate Strings("$1MJ\u0004-" ("write buffer"), w1187) -> (w1191:string)
                    n259 = VISA Write(VISA resource name=w1185, write buffer=w1191, error in (no error)=w1184) -> ()  [unwired: 3 out]
                  }
                }
              }
            }
            n260 = case shown="True" w1144 {
              tunnel: [w1221 w1228] -> w1156
              tunnel: w1158 -> [w1220 w1223]
              tunnel: w1117 -> [_ w1224]
              tunnel: w1116 -> [_ w1225]
              frame False {
                n261 = Add(x=0, y=w1220) -> (x+y=w1221:i32)
                n262 = Wait (ms)(milliseconds to wait=u32 500) -> ()  [unwired: 1 out]
              }
              frame True {
                n263 = VISA Write(VISA resource name=w1224, write buffer="$1MJ\u0004+\u0000\u0000<", error in (no error)=w1225) -> ()  [unwired: 3 out]
                n264 = Add(x=60, y=w1223) -> (x+y=w1228:i32)
              }
            }
            n265 = case shown="True" w1141 {
              tunnel: [w1211 w1214] -> w1155
              tunnel: w1157 -> [w1210 w1213]
              tunnel: w1117 -> [_ w1217]
              tunnel: w1116 -> [_ w1216]
              frame False {
                n266 = Add(x=0, y=w1210) -> (x+y=w1211:i32)
                n267 = Wait (ms)(milliseconds to wait=u32 500) -> ()  [unwired: 1 out]
              }
              frame True {
                n268 = Subtract(x=w1213, y=60 ("x")) -> (x-y=w1214:i32)
                n269 = VISA Write(VISA resource name=w1217, write buffer="$1MJ\u0004-\u0000\u0000<", error in (no error)=w1216) -> ()  [unwired: 3 out]
              }
            }
            n270 = for {
              N: 1 -> [_]
              tunnel: [w1163] -> w1120 mode=indexing
              n271 = local read "1"() -> (w1163:i32)
            }
            n272 = Index Array(array=w1120, index=0) -> (element=w1122:i32)
          }
          frame #2 {
            # "Нулевое положение"
            n273 = Add(x=w1247, y=w1248) -> (x+y=w1258:i32)
            n274 = Add(x=w1245, y=w1246) -> (x+y=w1260:i32)
            n275 = Add(x=w1260, y=w1258) -> (x+y=w1238:i32)
            n276 = Add(x=w1238, y=w1235) -> (x+y=w1237:i32)
            n277 = Not Equal?(x=w1237, y=0 ("x")) -> (x != y?=w1255:bool)
            n278 = And(x=w1255, y=w1257) -> (x .and. y?=w1262:bool)
            n279 = case shown="True" w1262 {
              tunnel: [w1296 w1319] -> w1234
              tunnel: w1245 -> [w1300 w1316]
              tunnel: [w1300 w1315] -> w1263
              tunnel: [w1299 w1314] -> w1261
              tunnel: w1237 -> [w1296 w1308]
              tunnel: [w1297 w1310] -> w1259
              tunnel: [w1298 w1307] -> w1254
              tunnel: w1246 -> [w1299 w1306]
              tunnel: w1253 -> [_ w1305]
              tunnel: w1252 -> [_ w1304]
              tunnel: w1247 -> [w1298 w1303]
              tunnel: w1248 -> [w1297 w1302]
              frame False {
              }
              frame True {
                n280 = Greater?(x=w1308, y=0) -> (0:w1309:bool)
                n281 = Multiply(x=w1302, y=0) -> (x*y=w1310:i32)
                n282 = Multiply(x=w1306, y=0) -> (x*y=w1314:i32)
                n283 = case shown="True" w1309 {
                  tunnel: w1308 -> [w1324 w1337]
                  tunnel: [0 0] -> w1319
                  tunnel: w1304 -> [w1321 w1334]
                  tunnel: w1305 -> [w1320 w1333]
                  frame False {
                    n284 = Multiply(x=w1324, y=-1) -> (x*y=w1322:i32)
                    n285 = Type Cast(type="", x=w1322) -> (*(type *) &x=w1328:string)
                    n286 = String Subset(string=w1328, offset (0)=1, length (rest)=3 ("length (rest)")) -> (substring=w1327:string)
                    n287 = Concatenate Strings("$1MJ\u0004+" ("write buffer"), w1327) -> (w1331:string)
                    n288 = VISA Write(VISA resource name=w1321, write buffer=w1331, error in (no error)=w1320) -> ()  [unwired: 3 out]
                  }
                  frame True {
                    n289 = Type Cast(type="", x=w1337) -> (*(type *) &x=w1340:string)
                    n290 = String Subset(string=w1340, offset (0)=1, length (rest)=3 ("length (rest)")) -> (substring=w1339:string)
                    n291 = Concatenate Strings("$1MJ\u0004-" ("write buffer"), w1339) -> (w1335:string)
                    n292 = VISA Write(VISA resource name=w1334, write buffer=w1335, error in (no error)=w1333) -> ()  [unwired: 3 out]
                  }
                }
                n293 = Multiply(x=w1303, y=0) -> (x*y=w1307:i32)
                n294 = Multiply(x=w1316, y=0) -> (x*y=w1315:i32)
                n295 = local write "1"(0 ("1")) -> ()
              }
            }
            "положение в мин 1" <- w1234
            n296 = Greater Or Equal?(x=w1234, y=0) -> (x >= y?=w1232:bool)
            n297 = Number To Decimal String(number=w1234, width (-)=i16 1) -> (decimal integer string=w1241:string)
            n298 = case shown="True" w1242 {
              tunnel: w1239 -> [w1264 w1271]
              tunnel: w1234 -> [_ w1272]
              tunnel: [w1264 w1270] -> w1236
              frame False {
              }
              frame True {
                n299 = Format Into String(w1272) -> (resulting string=w1268:string)  [unwired: 3 in, 1 out]
                n300 = local read "text2"() -> (w1267:string)
                n301 = local read "text3"() -> (w1266:string)
                n302 = local read "text4"() -> (w1265:string)
                n303 = Concatenate Strings(w1268, w1267, w1266, w1265) -> (w1269:string)
                n304 = Write to Text File(file (use dialog)=w1271, text=w1269) -> (refnum out=w1270:refnum<file>)  [unwired: 2 in, 2 out]
              }
            }
            n305 = case shown="False" w1232 {
              tunnel: w1234 -> [w1279 w1295]
              tunnel: [w1283 w1289] -> w1251
              tunnel: [w1273 w1287] -> w1249
              frame False {
                n306 = Multiply(x=-1, y=w1279) -> (x*y=w1278:i32)
                n307 = Quotient & Remainder(x=w1278, y=60) -> (x-y*floor(x/y)=w1282:i32, floor(x/y)=w1274:i32)
                n308 = Multiply(x=-1, y=w1274) -> (x*y=w1273:i32)
                n309 = Number To Decimal String(number=w1274) -> (decimal integer string=w1280:string)  [unwired: 1 in]
                n310 = Number To Decimal String(number=w1282) -> (decimal integer string=w1281:string)  [unwired: 1 in]
                n311 = Concatenate Strings("-" ("string"), w1280, "°" ("string"), w1281, "'" ("string")) -> (w1283:string)
              }
              frame True {
                n312 = Quotient & Remainder(x=w1295, y=60) -> (x-y*floor(x/y)=w1288:i32, floor(x/y)=w1287:i32)
                n313 = Number To Decimal String(number=w1288) -> (decimal integer string=w1290:string)  [unwired: 1 in]
                n314 = Number To Decimal String(number=w1287) -> (decimal integer string=w1291:string)  [unwired: 1 in]
                n315 = Concatenate Strings(w1291, "°" ("string"), w1290, "'" ("string")) -> (w1289:string)
              }
            }
            "положение шд" <- w1249
            "градусы минуты" <- w1251
            n316 = Concatenate Strings(w1241, "'" ("string")) -> (→"минуты":string)
          }
          frame #3 {
            # "Задача нуля"
            n317 = Or(x=w1345, y=w1346) -> (x .or. y?=w1344:bool)
            n318 = case shown="True" w1345 {
              tunnel: w1348 -> [_ w1358]
              tunnel: w1347 -> [_ w1357]
              frame False {
              }
              frame True {
                n319 = VISA Write(VISA resource name=w1358, write buffer="$1MS\u0001", error in (no error)=w1357) -> ()  [unwired: 3 out]
              }
            }
            n320 = case shown="True" w1344 {
              tunnel: [w1363 w1375] -> w1356
              tunnel: w1355 -> [w1363 w1376]
              tunnel: w1354 -> [w1362 w1372]
              tunnel: [w1362 w1371] -> w1353
              tunnel: [w1361 w1368] -> w1352
              tunnel: [w1360 w1367] -> w1351
              tunnel: w1350 -> [w1361 w1366]
              tunnel: w1349 -> [w1360 w1365]
              frame False {
              }
              frame True {
                n321 = Multiply(x=w1372, y=0) -> (x*y=w1371:i32)
                n322 = Multiply(x=w1376, y=0) -> (x*y=w1375:i32)
                n323 = local write "1"(0 ("1")) -> ()
                n324 = Multiply(x=w1365, y=0) -> (x*y=w1367:i32)
                n325 = Multiply(x=w1366, y=0) -> (x*y=w1368:i32)
              }
            }
          }
        }
        n326 = flat-sequence {
          tunnel: w124 -> [w273]
          tunnel: w125 -> [w274]
          tunnel: [w274] -> w146
          tunnel: [w273] -> w145
          tunnel: ["Вращение по градусам +  4"] -> w144
          tunnel: ["Вращение по градусам -  4"] -> w143
          tunnel: ["Вернуться в нулевое положение 4"] -> w142
          tunnel: ["Задать текущее положение нулевым 4"] -> w141
          tunnel: ["Установка минут 4"] -> w140
          tunnel: ["Stop двигатель 4"] -> w95
          tunnel: w146 -> [w276]
          tunnel: w145 -> [w275]
          tunnel: [w321] -> w139
          tunnel: w122 -> [w318]
          tunnel: w120 -> [w320]
          tunnel: [w319] -> w138
          tunnel: w118 -> [w317]
          tunnel: w116 -> [w316]
          tunnel: w144 -> [w302]
          tunnel: w143 -> [w301]
          tunnel: [w315] -> w137
          tunnel: [w314] -> w136
          tunnel: [w299] -> w135
          tunnel: w142 -> [w299]
          tunnel: [w275] -> w134
          tunnel: [w276] -> w133
          tunnel: [w298] -> w132
          tunnel: w141 -> [w298]
          tunnel: w140 -> [w292]
          tunnel: [w282] -> w131
          tunnel: [w277] -> w96
          tunnel: w95 -> [w277]
          tunnel: [w276] -> w93
          tunnel: [w275] -> w92
          tunnel: w139 -> [w406]
          tunnel: w138 -> [w407]
          tunnel: [w422] -> w130
          tunnel: [w420] -> w129
          tunnel: w137 -> [w408]
          tunnel: w136 -> [w409]
          tunnel: [w413] -> w128
          tunnel: [w418] -> w127
          tunnel: w135 -> [w416]
          tunnel: w134 -> [w412]
          tunnel: w133 -> [w411]
          tunnel: w132 -> [w410]
          tunnel: [w410] -> w126
          tunnel: w131 -> [w397]
          tunnel: [w390] -> w97
          tunnel: w96 -> [w390]
          tunnel: [w389] -> w94
          tunnel: w93 -> [w389]
          tunnel: w92 -> [w388]
          tunnel: [w388] -> w91
          tunnel: [w506] -> w121
          tunnel: [w503] -> w119
          tunnel: w130 -> [w505]
          tunnel: w129 -> [w504]
          tunnel: [w502] -> w117
          tunnel: [w501] -> w115
          tunnel: w128 -> [w500]
          tunnel: w127 -> [w499]
          tunnel: w126 -> [w497]
          tunnel: w97 -> [w498]
          tunnel: w94 -> [w495]
          tunnel: w91 -> [w494]
          frame #0 {
            n327 = Wait Until Next ms Multiple(millisecond multiple=u32 300) -> ()  [unwired: 1 out]
          }
          frame #1 {
            # "Остановка двигателя"
            n328 = Greater?(x="Минуты 4", y=0) -> (0:w290:bool)
            n329 = Not Equal?(x="Минуты 4", y=0) -> (x != y?=w289:bool)
            n330 = local read "положение в мин 4"() -> (w283:i32)
            n331 = Add(x="Минуты 4", y=w283) -> (x+y=w312:i32)
            n332 = Add(x="Минуты 4", y=w283) -> (x+y=w285:i32)
            n333 = Not Equal?(x="Минуты 4", y=0) -> (x != y?=w287:bool)
            n334 = Add(x=w283, y=60) -> (x+y=w307:i32)
            n335 = Subtract(x=w283, y=60) -> (x-y=w295:i32)
            n336 = Not(x=w290) -> (.not. x?=w291:bool)
            n337 = Greater Or Equal?(x=w285, y=-600) -> (x >= y?=w286:bool)
            n338 = Less Or Equal?(x=w312, y=11400) -> (x <= y?=w288:bool)
            n339 = Less Or Equal?(x=w307, y=11390) -> (x <= y?=w304:bool)
            n340 = Greater Or Equal?(x=w295, y=-590) -> (x >= y?=w296:bool)
            n341 = Compound Arithmetic op=AND(w291, w287, w286) -> (w308:bool)
            n342 = And(x=w302, y=w304) -> (x .and. y?=w303:bool)
            n343 = And(x=w301, y=w296) -> (x .and. y?=w300:bool)
            n344 = Compound Arithmetic op=AND(w290, w289, w288) -> (w310:bool)
            n345 = case shown="True" w292 {
              tunnel: [w324 w333] -> w321
              tunnel: w320 -> [w323 w332]
              tunnel: [w323 w331] -> w319
              tunnel: w318 -> [w324 w330]
              tunnel: w310 -> [_ w329]
              tunnel: w308 -> [_ w328]
              tunnel: w275 -> [_ w327]
              tunnel: w276 -> [_ w326]
              tunnel: "Минуты 4" -> [_ w325]
              frame False {
              }
              frame True {
                n346 = case shown="True" w329 {
                  tunnel: [w354 w360] -> w333
                  tunnel: w330 -> [w353 w359]
                  tunnel: w327 -> [_ w358]
                  tunnel: w326 -> [_ w357]
                  tunnel: w325 -> [_ w356]
                  frame False {
                    n347 = Add(x=0, y=w353) -> (x+y=w354:i32)
                    n348 = Wait (ms)(milliseconds to wait=u32 500) -> ()  [unwired: 1 out]
                  }
                  frame True {
                    n349 = Type Cast(type="", x=w356) -> (*(type *) &x=w363:string)
                    n350 = Add(x=w356, y=w359) -> (x+y=w360:i32)
                    n351 = String Subset(string=w363, offset (0)=1, length (rest)=3 ("length (rest)")) -> (substring=w362:string)
                    n352 = Concatenate Strings("$4MJ\u0004+" ("write buffer"), w362) -> (w366:string)
                    n353 = VISA Write(VISA resource name=w357, write buffer=w366, error in (no error)=w358) -> ()  [unwired: 3 out]
                  }
                }
                n354 = case shown="True" w328 {
                  tunnel: [w336 w342] -> w331
                  tunnel: w332 -> [w335 w341]
                  tunnel: w326 -> [_ w344]
                  tunnel: w327 -> [_ w343]
                  tunnel: w325 -> [_ w338]
                  frame False {
                    n355 = Add(x=0, y=w335) -> (x+y=w336:i32)
                    n356 = Wait (ms)(milliseconds to wait=u32 500) -> ()  [unwired: 1 out]
                  }
                  frame True {
                    n357 = Multiply(x=w338, y=-1) -> (x*y=w340:i32)
                    n358 = Type Cast(type="", x=w340) -> (*(type *) &x=w347:string)
                    n359 = Add(x=w341, y=w338) -> (x+y=w342:i32)
                    n360 = String Subset(string=w347, offset (0)=1, length (rest)=3 ("length (rest)")) -> (substring=w346:string)
                    n361 = Concatenate Strings("$4MJ\u0004-" ("write buffer"), w346) -> (w350:string)
                    n362 = VISA Write(VISA resource name=w344, write buffer=w350, error in (no error)=w343) -> ()  [unwired: 3 out]
                  }
                }
              }
            }
            n363 = case shown="True" w303 {
              tunnel: [w380 w387] -> w315
              tunnel: w317 -> [w379 w382]
              tunnel: w276 -> [_ w383]
              tunnel: w275 -> [_ w384]
              frame False {
                n364 = Add(x=0, y=w379) -> (x+y=w380:i32)
                n365 = Wait (ms)(milliseconds to wait=u32 500) -> ()  [unwired: 1 out]
              }
              frame True {
                n366 = VISA Write(VISA resource name=w383, write buffer="$4MJ\u0004+\u0000\u0000<", error in (no error)=w384) -> ()  [unwired: 3 out]
                n367 = Add(x=60, y=w382) -> (x+y=w387:i32)
              }
            }
            n368 = case shown="True" w300 {
              tunnel: [w370 w373] -> w314
              tunnel: w316 -> [w369 w372]
              tunnel: w276 -> [_ w376]
              tunnel: w275 -> [_ w375]
              frame False {
                n369 = Add(x=0, y=w369) -> (x+y=w370:i32)
                n370 = Wait (ms)(milliseconds to wait=u32 500) -> ()  [unwired: 1 out]
              }
              frame True {
                n371 = Subtract(x=w372, y=60 ("x")) -> (x-y=w373:i32)
                n372 = VISA Write(VISA resource name=w376, write buffer="$4MJ\u0004-\u0000\u0000<", error in (no error)=w375) -> ()  [unwired: 3 out]
              }
            }
            n373 = for {
              N: 1 -> [_]
              tunnel: [w322] -> w280 mode=indexing
              n374 = local read "4"() -> (w322:i32)
            }
            n375 = Index Array(array=w280, index=0) -> (element=w282:i32)
          }
          frame #2 {
            # "Нулевое положение"
            n376 = Add(x=w408, y=w409) -> (x+y=w417:i32)
            n377 = Add(x=w406, y=w407) -> (x+y=w419:i32)
            n378 = Add(x=w419, y=w417) -> (x+y=w402:i32)
            n379 = Add(x=w402, y=w397) -> (x+y=w401:i32)
            n380 = Not Equal?(x=w401, y=0 ("x")) -> (x != y?=w414:bool)
            n381 = And(x=w414, y=w416) -> (x .and. y?=w421:bool)
            n382 = case shown="True" w421 {
              tunnel: [w446 w469] -> w393
              tunnel: w406 -> [w450 w466]
              tunnel: [w450 w465] -> w422
              tunnel: [w449 w464] -> w420
              tunnel: w401 -> [w446 w458]
              tunnel: [w447 w460] -> w418
              tunnel: [w448 w457] -> w413
              tunnel: w407 -> [w449 w456]
              tunnel: w412 -> [_ w455]
              tunnel: w411 -> [_ w454]
              tunnel: w408 -> [w448 w453]
              tunnel: w409 -> [w447 w452]
              frame False {
              }
              frame True {
                n383 = Greater?(x=w458, y=0) -> (0:w459:bool)
                n384 = Multiply(x=w452, y=0) -> (x*y=w460:i32)
                n385 = Multiply(x=w456, y=0) -> (x*y=w464:i32)
                n386 = case shown="True" w459 {
                  tunnel: w458 -> [w474 w487]
                  tunnel: [0 0] -> w469
                  tunnel: w454 -> [w471 w484]
                  tunnel: w455 -> [w470 w483]
                  frame False {
                    n387 = Multiply(x=w474, y=-1) -> (x*y=w472:i32)
                    n388 = Type Cast(type="", x=w472) -> (*(type *) &x=w478:string)
                    n389 = String Subset(string=w478, offset (0)=1, length (rest)=3 ("length (rest)")) -> (substring=w477:string)
                    n390 = Concatenate Strings("$4MJ\u0004+" ("write buffer"), w477) -> (w481:string)
                    n391 = VISA Write(VISA resource name=w471, write buffer=w481, error in (no error)=w470) -> ()  [unwired: 3 out]
                  }
                  frame True {
                    n392 = Type Cast(type="", x=w487) -> (*(type *) &x=w490:string)
                    n393 = String Subset(string=w490, offset (0)=1, length (rest)=3 ("length (rest)")) -> (substring=w489:string)
                    n394 = Concatenate Strings("$4MJ\u0004-" ("write buffer"), w489) -> (w485:string)
                    n395 = VISA Write(VISA resource name=w484, write buffer=w485, error in (no error)=w483) -> ()  [unwired: 3 out]
                  }
                }
                n396 = Multiply(x=w453, y=0) -> (x*y=w457:i32)
                n397 = Multiply(x=w466, y=0) -> (x*y=w465:i32)
                n398 = local write "4"(0 ("4")) -> ()
              }
            }
            "положение в мин 4" <- w393
            n399 = Greater Or Equal?(x=w393, y=0) -> (x >= y?=w391:bool)
            n400 = Number To Decimal String(number=w393, width (-)=i16 1) -> (decimal integer string=w404:string)
            n401 = case shown="False" w391 {
              tunnel: w393 -> [w429 w445]
              tunnel: [w433 w439] -> w395
              tunnel: [w423 w437] -> w396
              frame False {
                n402 = Multiply(x=-1, y=w429) -> (x*y=w428:i32)
                n403 = Quotient & Remainder(x=w428, y=60) -> (x-y*floor(x/y)=w432:i32, floor(x/y)=w424:i32)
                n404 = Multiply(x=-1, y=w424) -> (x*y=w423:i32)
                n405 = Number To Decimal String(number=w424) -> (decimal integer string=w430:string)  [unwired: 1 in]
                n406 = Number To Decimal String(number=w432) -> (decimal integer string=w431:string)  [unwired: 1 in]
                n407 = Concatenate Strings("-" ("string"), w430, "°" ("string"), w431, "'" ("string")) -> (w433:string)
              }
              frame True {
                n408 = Quotient & Remainder(x=w445, y=60) -> (x-y*floor(x/y)=w438:i32, floor(x/y)=w437:i32)
                n409 = Number To Decimal String(number=w438) -> (decimal integer string=w440:string)  [unwired: 1 in]
                n410 = Number To Decimal String(number=w437) -> (decimal integer string=w441:string)  [unwired: 1 in]
                n411 = Concatenate Strings(w441, "°" ("string"), w440, "'" ("string")) -> (w439:string)
              }
            }
            "положение шд 4" <- w396
            "текущее положение 4" <- w395
            n412 = Concatenate Strings(w404, "'" ("string")) -> (→"положение в минутах 4":string)
            n413 = Format Into String(w393) -> (resulting string=w399:string)  [unwired: 3 in, 1 out]
            n414 = call <vilib>:"Space Constant.vi"() -> ("String"=w398:string)
            n415 = Concatenate Strings(w398, w399) -> (→"text4":string)
          }
          frame #3 {
            # "Задача нуля"
            n416 = case shown="True" w498 {
              tunnel: w495 -> [_ w508]
              tunnel: w494 -> [_ w507]
              frame False {
              }
              frame True {
                n417 = Wait (ms)(milliseconds to wait=u32 500) -> ()  [unwired: 1 out]
                n418 = VISA Write(VISA resource name=w508, write buffer="$4MS\u0001", error in (no error)=w507) -> ()  [unwired: 3 out]
              }
            }
            n419 = Or(x=w497, y=w498) -> (x .or. y?=w496:bool)
            n420 = case shown="True" w496 {
              tunnel: [w514 w526] -> w506
              tunnel: w505 -> [w514 w527]
              tunnel: w504 -> [w513 w523]
              tunnel: [w513 w522] -> w503
              tunnel: [w512 w519] -> w502
              tunnel: [w511 w518] -> w501
              tunnel: w500 -> [w512 w517]
              tunnel: w499 -> [w511 w516]
              frame False {
              }
              frame True {
                n421 = Multiply(x=w523, y=0) -> (x*y=w522:i32)
                n422 = Multiply(x=w527, y=0) -> (x*y=w526:i32)
                n423 = local write "4"(0 ("4")) -> ()
                n424 = Multiply(x=w516, y=0) -> (x*y=w518:i32)
                n425 = Multiply(x=w517, y=0) -> (x*y=w519:i32)
              }
            }
          }
        }
        n426 = case shown="True" "Блокировать трубку №2" {
          frame False {
            n427 = property on="Stop двигатель 2" class="Bool"("DisabledEnum"=T3."Enabled" ("Disabled")) -> ()  [unwired: 2 in, 2 out]
            n428 = property on="Вернуться в нулевое положение 2" class="Bool"("DisabledEnum"=T3."Enabled" ("Disabled")) -> ()  [unwired: 2 in, 2 out]
            n429 = property on="Вращение по градусам +  2" class="Bool"("DisabledEnum"=T3."Enabled" ("Disabled")) -> ()  [unwired: 2 in, 2 out]
            n430 = property on="текущее положение 2" class="Str"("DisabledEnum"=T3."Enabled" ("Disabled")) -> ()  [unwired: 2 in, 2 out]
            n431 = property on="Установка минут 2" class="Bool"("DisabledEnum"=T3."Enabled" ("Disabled")) -> ()  [unwired: 2 in, 2 out]
            n432 = property on="Вращение по градусам -  2" class="Bool"("DisabledEnum"=T3."Enabled" ("Disabled")) -> ()  [unwired: 2 in, 2 out]
            n433 = property on="Задать текущее положение нулевым 2" class="Bool"("DisabledEnum"=T3."Enabled" ("Disabled")) -> ()  [unwired: 2 in, 2 out]
            n434 = property on="Минуты 2" class="DigNum (strict)"("DisabledEnum"=T3."Enabled" ("Disabled")) -> ()  [unwired: 2 in, 2 out]
            n435 = property on="положение шд 2" class="Knob (strict)"("DisabledEnum"=T3."Enabled" ("Disabled")) -> ()  [unwired: 2 in, 2 out]
            n436 = property on="положение в минутах 2" class="Str"("DisabledEnum"=T3."Enabled" ("Disabled")) -> ()  [unwired: 2 in, 2 out]
          }
          frame True {
            n437 = property on="Вернуться в нулевое положение 2" class="Bool"("DisabledEnum"=T3."Disabled and Grayed Out" ("Disabled")) -> ()  [unwired: 2 in, 2 out]
            n438 = property on="положение шд 2" class="Knob (strict)"("DisabledEnum"=T3."Disabled and Grayed Out" ("Disabled")) -> ()  [unwired: 2 in, 2 out]
            n439 = property on="текущее положение 2" class="Str"("DisabledEnum"=T3."Disabled and Grayed Out" ("Disabled")) -> ()  [unwired: 2 in, 2 out]
            n440 = property on="Stop двигатель 2" class="Bool"("DisabledEnum"=T3."Disabled and Grayed Out" ("Disabled")) -> ()  [unwired: 2 in, 2 out]
            n441 = property on="Вращение по градусам +  2" class="Bool"("DisabledEnum"=T3."Disabled and Grayed Out" ("Disabled")) -> ()  [unwired: 2 in, 2 out]
            n442 = property on="Вращение по градусам -  2" class="Bool"("DisabledEnum"=T3."Disabled and Grayed Out" ("Disabled")) -> ()  [unwired: 2 in, 2 out]
            n443 = property on="Задать текущее положение нулевым 2" class="Bool"("DisabledEnum"=T3."Disabled and Grayed Out" ("Disabled")) -> ()  [unwired: 2 in, 2 out]
            n444 = property on="Минуты 2" class="DigNum (strict)"("DisabledEnum"=T3."Disabled and Grayed Out" ("Disabled")) -> ()  [unwired: 2 in, 2 out]
            n445 = property on="Установка минут 2" class="Bool"("DisabledEnum"=T3."Disabled and Grayed Out" ("Disabled")) -> ()  [unwired: 2 in, 2 out]
            n446 = property on="положение в минутах 2" class="Str"("DisabledEnum"=T3."Disabled and Grayed Out" ("Disabled")) -> ()  [unwired: 2 in, 2 out]
          }
        }
        n447 = case shown="False" "Блокировать зеркало №1" {
          frame False {
            n448 = property on="Stop двигатель" class="Bool"("DisabledEnum"=T3."Enabled" ("Disabled")) -> ()  [unwired: 2 in, 2 out]
            n449 = property on="Вернуться в нулевое положение" class="Bool"("DisabledEnum"=T3."Enabled" ("Disabled")) -> ()  [unwired: 2 in, 2 out]
            n450 = property on="Вращение по градусам +" class="Bool"("DisabledEnum"=T3."Enabled" ("Disabled")) -> ()  [unwired: 2 in, 2 out]
            n451 = property on="градусы минуты" class="Str"("DisabledEnum"=T3."Enabled" ("Disabled")) -> ()  [unwired: 2 in, 2 out]
            n452 = property on="Установка минут" class="Bool"("DisabledEnum"=T3."Enabled" ("Disabled")) -> ()  [unwired: 2 in, 2 out]
            n453 = property on="Вращение по градусам -" class="Bool (strict)"("DisabledEnum"=T3."Enabled" ("Disabled")) -> ()  [unwired: 2 in, 2 out]
            n454 = property on="Задать текущее положение нулевым" class="Bool"("DisabledEnum"=T3."Enabled" ("Disabled")) -> ()  [unwired: 2 in, 2 out]
            n455 = property on="Минуты" class="DigNum (strict)"("DisabledEnum"=T3."Enabled" ("Disabled")) -> ()  [unwired: 2 in, 2 out]
            n456 = property on="положение шд" class="Knob (strict)"("DisabledEnum"=T3."Enabled" ("Disabled")) -> ()  [unwired: 2 in, 2 out]
            n457 = property on="минуты" class="Str"("DisabledEnum"=T3."Enabled" ("Disabled")) -> ()  [unwired: 2 in, 2 out]
          }
          frame True {
            n458 = property on="Вернуться в нулевое положение" class="Bool"("DisabledEnum"=T3."Disabled and Grayed Out" ("Disabled")) -> ()  [unwired: 2 in, 2 out]
            n459 = property on="положение шд" class="Knob (strict)"("DisabledEnum"=T3."Disabled and Grayed Out" ("Disabled")) -> ()  [unwired: 2 in, 2 out]
            n460 = property on="градусы минуты" class="Str"("DisabledEnum"=T3."Disabled and Grayed Out" ("Disabled")) -> ()  [unwired: 2 in, 2 out]
            n461 = property on="Stop двигатель" class="Bool"("DisabledEnum"=T3."Disabled and Grayed Out" ("Disabled")) -> ()  [unwired: 2 in, 2 out]
            n462 = property on="Вращение по градусам +" class="Bool"("DisabledEnum"=T3."Disabled and Grayed Out" ("Disabled")) -> ()  [unwired: 2 in, 2 out]
            n463 = property on="Вращение по градусам -" class="Bool (strict)"("DisabledEnum"=T3."Disabled and Grayed Out" ("Disabled")) -> ()  [unwired: 2 in, 2 out]
            n464 = property on="Задать текущее положение нулевым" class="Bool"("DisabledEnum"=T3."Disabled and Grayed Out" ("Disabled")) -> ()  [unwired: 2 in, 2 out]
            n465 = property on="Минуты" class="DigNum (strict)"("DisabledEnum"=T3."Disabled and Grayed Out" ("Disabled")) -> ()  [unwired: 2 in, 2 out]
            n466 = property on="Установка минут" class="Bool"("DisabledEnum"=T3."Disabled and Grayed Out" ("Disabled")) -> ()  [unwired: 2 in, 2 out]
            n467 = property on="минуты" class="Str"("DisabledEnum"=T3."Disabled and Grayed Out" ("Disabled")) -> ()  [unwired: 2 in, 2 out]
          }
        }
        n468 = case shown="False" "Блокировать стол №3 2" {
          frame False {
            n469 = property on="Stop двигатель 4" class="Bool"("DisabledEnum"=T3."Enabled" ("Disabled")) -> ()  [unwired: 2 in, 2 out]
            n470 = property on="Вернуться в нулевое положение 4" class="Bool"("DisabledEnum"=T3."Enabled" ("Disabled")) -> ()  [unwired: 2 in, 2 out]
            n471 = property on="Вращение по градусам +  4" class="Bool"("DisabledEnum"=T3."Enabled" ("Disabled")) -> ()  [unwired: 2 in, 2 out]
            n472 = property on="текущее положение 4" class="Str"("DisabledEnum"=T3."Enabled" ("Disabled")) -> ()  [unwired: 2 in, 2 out]
            n473 = property on="Установка минут 4" class="Bool"("DisabledEnum"=T3."Enabled" ("Disabled")) -> ()  [unwired: 2 in, 2 out]
            n474 = property on="Вращение по градусам -  4" class="Bool"("DisabledEnum"=T3."Enabled" ("Disabled")) -> ()  [unwired: 2 in, 2 out]
            n475 = property on="Задать текущее положение нулевым 4" class="Bool"("DisabledEnum"=T3."Enabled" ("Disabled")) -> ()  [unwired: 2 in, 2 out]
            n476 = property on="Минуты 4" class="DigNum (strict)"("DisabledEnum"=T3."Enabled" ("Disabled")) -> ()  [unwired: 2 in, 2 out]
            n477 = property on="положение шд 4" class="Knob (strict)"("DisabledEnum"=T3."Enabled" ("Disabled")) -> ()  [unwired: 2 in, 2 out]
            n478 = property on="положение в минутах 4" class="Str"("DisabledEnum"=T3."Enabled" ("Disabled")) -> ()  [unwired: 2 in, 2 out]
          }
          frame True {
            n479 = property on="Вернуться в нулевое положение 4" class="Bool"("DisabledEnum"=T3."Disabled and Grayed Out" ("Disabled")) -> ()  [unwired: 2 in, 2 out]
            n480 = property on="положение шд 4" class="Knob (strict)"("DisabledEnum"=T3."Disabled and Grayed Out" ("Disabled")) -> ()  [unwired: 2 in, 2 out]
            n481 = property on="текущее положение 4" class="Str"("DisabledEnum"=T3."Disabled and Grayed Out" ("Disabled")) -> ()  [unwired: 2 in, 2 out]
            n482 = property on="Stop двигатель 4" class="Bool"("DisabledEnum"=T3."Disabled and Grayed Out" ("Disabled")) -> ()  [unwired: 2 in, 2 out]
            n483 = property on="Вращение по градусам +  4" class="Bool"("DisabledEnum"=T3."Disabled and Grayed Out" ("Disabled")) -> ()  [unwired: 2 in, 2 out]
            n484 = property on="Вращение по градусам -  4" class="Bool"("DisabledEnum"=T3."Disabled and Grayed Out" ("Disabled")) -> ()  [unwired: 2 in, 2 out]
            n485 = property on="Задать текущее положение нулевым 4" class="Bool"("DisabledEnum"=T3."Disabled and Grayed Out" ("Disabled")) -> ()  [unwired: 2 in, 2 out]
            n486 = property on="Минуты 4" class="DigNum (strict)"("DisabledEnum"=T3."Disabled and Grayed Out" ("Disabled")) -> ()  [unwired: 2 in, 2 out]
            n487 = property on="Установка минут 4" class="Bool"("DisabledEnum"=T3."Disabled and Grayed Out" ("Disabled")) -> ()  [unwired: 2 in, 2 out]
            n488 = property on="положение в минутах 4" class="Str"("DisabledEnum"=T3."Disabled and Grayed Out" ("Disabled")) -> ()  [unwired: 2 in, 2 out]
          }
        }
        n489 = case shown="False" "Блокировать стол №3" {
          frame False {
            n490 = property on="Stop двигатель 3" class="Bool (strict)"("DisabledEnum"=T3."Enabled" ("Disabled")) -> ()  [unwired: 2 in, 2 out]
            n491 = property on="Вернуться в нулевое положение 3" class="Bool"("DisabledEnum"=T3."Enabled" ("Disabled")) -> ()  [unwired: 2 in, 2 out]
            n492 = property on="Вращение по градусам +  3" class="Bool"("DisabledEnum"=T3."Enabled" ("Disabled")) -> ()  [unwired: 2 in, 2 out]
            n493 = property on="текущее положение 3" class="Str"("DisabledEnum"=T3."Enabled" ("Disabled")) -> ()  [unwired: 2 in, 2 out]
            n494 = property on="Установка минут 3" class="Bool"("DisabledEnum"=T3."Enabled" ("Disabled")) -> ()  [unwired: 2 in, 2 out]
            n495 = property on="Вращение по градусам -  3" class="Bool"("DisabledEnum"=T3."Enabled" ("Disabled")) -> ()  [unwired: 2 in, 2 out]
            n496 = property on="Задать текущее положение нулевым 3" class="Bool"("DisabledEnum"=T3."Enabled" ("Disabled")) -> ()  [unwired: 2 in, 2 out]
            n497 = property on="Минуты 3" class="DigNum (strict)"("DisabledEnum"=T3."Enabled" ("Disabled")) -> ()  [unwired: 2 in, 2 out]
            n498 = property on="положение шд 3" class="Knob (strict)"("DisabledEnum"=T3."Enabled" ("Disabled")) -> ()  [unwired: 2 in, 2 out]
            n499 = property on="положение в минутах 3" class="Str"("DisabledEnum"=T3."Enabled" ("Disabled")) -> ()  [unwired: 2 in, 2 out]
          }
          frame True {
            n500 = property on="Вернуться в нулевое положение 3" class="Bool"("DisabledEnum"=T3."Disabled and Grayed Out" ("Disabled")) -> ()  [unwired: 2 in, 2 out]
            n501 = property on="положение шд 3" class="Knob (strict)"("DisabledEnum"=T3."Disabled and Grayed Out" ("Disabled")) -> ()  [unwired: 2 in, 2 out]
            n502 = property on="текущее положение 3" class="Str"("DisabledEnum"=T3."Disabled and Grayed Out" ("Disabled")) -> ()  [unwired: 2 in, 2 out]
            n503 = property on="Stop двигатель 3" class="Bool (strict)"("DisabledEnum"=T3."Disabled and Grayed Out" ("Disabled")) -> ()  [unwired: 2 in, 2 out]
            n504 = property on="Вращение по градусам +  3" class="Bool"("DisabledEnum"=T3."Disabled and Grayed Out" ("Disabled")) -> ()  [unwired: 2 in, 2 out]
            n505 = property on="Вращение по градусам -  3" class="Bool"("DisabledEnum"=T3."Disabled and Grayed Out" ("Disabled")) -> ()  [unwired: 2 in, 2 out]
            n506 = property on="Задать текущее положение нулевым 3" class="Bool"("DisabledEnum"=T3."Disabled and Grayed Out" ("Disabled")) -> ()  [unwired: 2 in, 2 out]
            n507 = property on="Минуты 3" class="DigNum (strict)"("DisabledEnum"=T3."Disabled and Grayed Out" ("Disabled")) -> ()  [unwired: 2 in, 2 out]
            n508 = property on="Установка минут 3" class="Bool"("DisabledEnum"=T3."Disabled and Grayed Out" ("Disabled")) -> ()  [unwired: 2 in, 2 out]
            n509 = property on="положение в минутах 3" class="Str"("DisabledEnum"=T3."Disabled and Grayed Out" ("Disabled")) -> ()  [unwired: 2 in, 2 out]
          }
        }
      }
      n510 = Close File(refnum=w86) -> ()  [unwired: 1 in, 2 out]
    }
  }
